vi "exportGraphsToPDF.Tangents XYGraph.vi"(7 "path":path, 8 "error in (no error)":errorcluster, 9 "Armpressure":dbl, 10 "Red Graph":refnum<vi>, 11 "Blue Graph":refnum<vi>) -> (0 "error out":errorcluster, 3 "output cluster":cluster{dbl, dbl, dbl, dbl})   [LabVIEW 2013, in "main.lvlib"]
uses:
  main.lvlib
  Controls/Combobox Filename.ctl
  <userlib>/_OpenG.lib/file/file.llb/File Exists - Scalar__ogtk.vi
  <vilib>/Utility/file.llb/Read From Spreadsheet File (DBL).vi
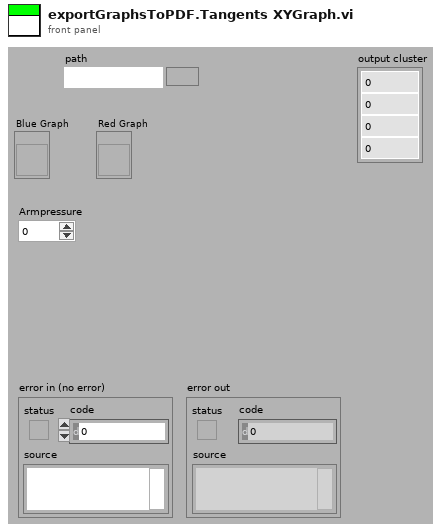
[diagram p1: front panel]
types:
  T1 = typedef "main.lvlib/Combobox Filename.ctl" = string
  T2 = cluster{dbl, dbl, "Armpressure":dbl, "Armpressure":dbl}
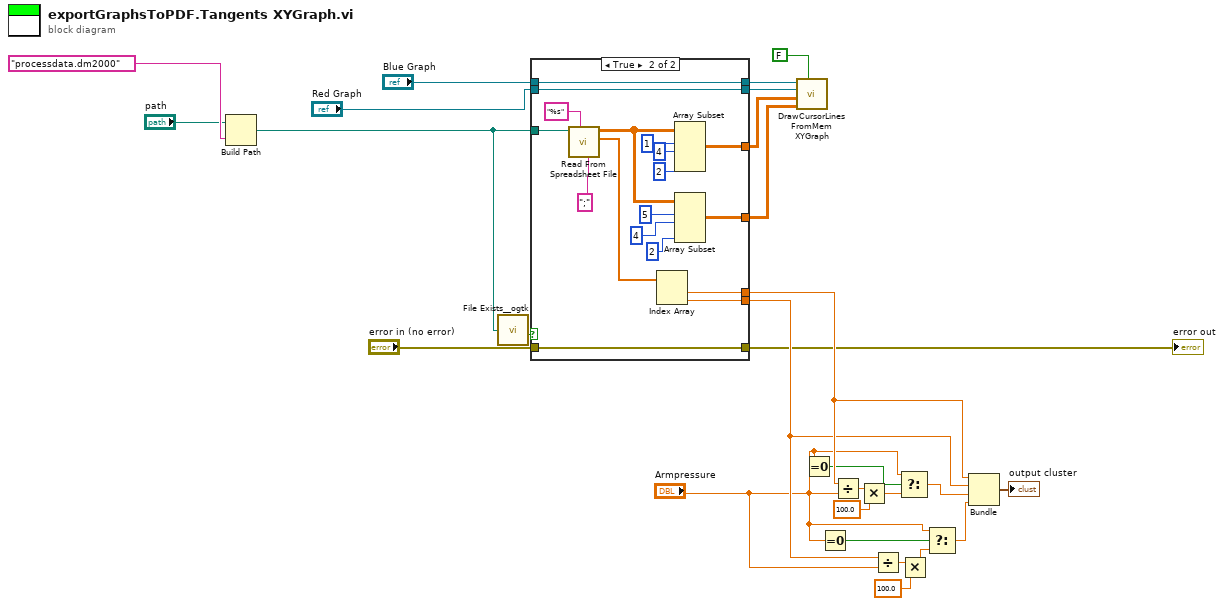
[diagram p0: block diagram]
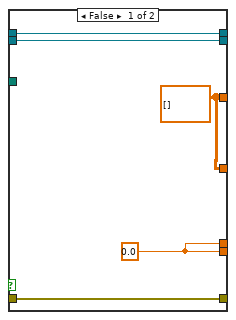
[diagram p2: hidden frame]
diagram:
  n1 = Build Path(base path="path", name or relative path=T1 "processdata.dm2000" ("FileName")) -> (appended path=w27:path)
  n2 = call-poly <userlib>:"File Exists__ogtk.vi"("file path"=w27) -> ("exists"=w23:bool)  [unwired: 6 in, 1 out]
  n3 = case shown="True" w23 {
    tunnel: w27 -> [_ w47]
    tunnel: [w32 w46] -> w14
    tunnel: [w32 w45] -> w17
    tunnel: [w31 w41] -> w21
    tunnel: [w31 w39] -> w22
    tunnel: [w30 w35] -> w25
    tunnel: "Blue Graph" -> [w30 w35]
    tunnel: "Red Graph" -> [w29 w34]
    tunnel: [w29 w34] -> w26
    tunnel: "error in (no error)" -> [w28 w33]
    tunnel: [w28 w33] -> w6
    frame False {
      w31 = dbl[][] []
      w32 = 0.0
    }
    frame True {
      n4 = call-poly <vilib>:"Read From Spreadsheet File.vi"("delimiter (\\t)"=";" ("delimiter (\\t)"), "format (%.3f)"="%s", "file path (dialog if empty)"=w47) -> ("first row"=w48:dbl[], "all rows"=w40:dbl[][])  [unwired: 4 in, 3 out]
      n5 = Index Array(array=w48) -> (element #1=w45:dbl, element #2=w46:dbl)  [unwired: 2 in]
      n6 = Array Subset(array=w40, index (row)=1 ("index"), length (row)=4 ("length"), length (col)=2 ("length")) -> (w41:dbl[][])  [unwired: 1 in]
      n7 = Array Subset(array=w40, index (row)=5 ("index"), length (row)=4 ("length"), length (col)=2 ("length")) -> (w39:dbl[][])  [unwired: 1 in]
    }
  }
  "error out" <- w6
  n8 = call "DrawCursorLinesFromMem XYGraph.vi"("CursorMode"=FALSE, "RedPositionArray"=w22, "BluePositionArray"=w21, "Red"=w26, "Blue"=w25) -> ()  [unwired: 7 in]
  n9 = Equal To 0?(x="Armpressure") -> (x = 0?=w12:bool)
  n10 = Equal To 0?(x="Armpressure") -> (x = 0?=w9:bool)
  n11 = Divide(x=w17, y="Armpressure") -> (x/y=w19:dbl)
  n12 = Multiply(x=w19, y=100.0) -> (x*y=w11:dbl)
  n13 = Divide(x=w14, y="Armpressure") -> (x/y=w16:dbl)
  n14 = Select(t="Armpressure", s=w12, f=w11) -> (s? t:f=w10:dbl)
  n15 = Multiply(x=w16, y=100.0) -> (x*y=w8:dbl)
  n16 = Select(t="Armpressure", s=w9, f=w8) -> (s? t:f=w7:dbl)
  n17 = Bundle(w17, w14, "Armpressure"=w10, "Armpressure"=w7) -> (→"output cluster":T2)  [unwired: 1 in]
